vi "JamesPIDTEST.vi"() -> ()   [LabVIEW 2014]
uses:
  <vilib>/Rock Robotics/WPI/Solenoid/WPI_SolenoidValue.ctl
  Robot Global Data.vi
  <vilib>/addons/control/pid/NI_PID_pid.lvlib
  <vilib>/addons/control/pid/pid.llb/PID Advanced (DBL).vi
panel:
  out "Setpoint":dbl
  in  "setpoint range":cluster{"setpoint high":dbl, "setpoint low":dbl}={"setpoint high"=100.0, "setpoint low"=0.0}
  out "output":dbl format="%.2f"
  out "Brake":bool
  in  "proportional gain (Kc)":dbl step=0.01
  in  "integral time (Ti, min)":dbl step=0.01
  in  "derivative time (Td, min)":dbl step=0.01
  in  "dt (s)":dbl=-1.0 format="%.3f"
  in  "SetPoint":dbl(slide) scale=3.7..4.5
  out "dx/dt":dbl format="%.3f"
  out "Grabber":bool
  out "Turn on Brake":bool
  out "Delay?":bool
  out "VoltageDiff Valid?":bool
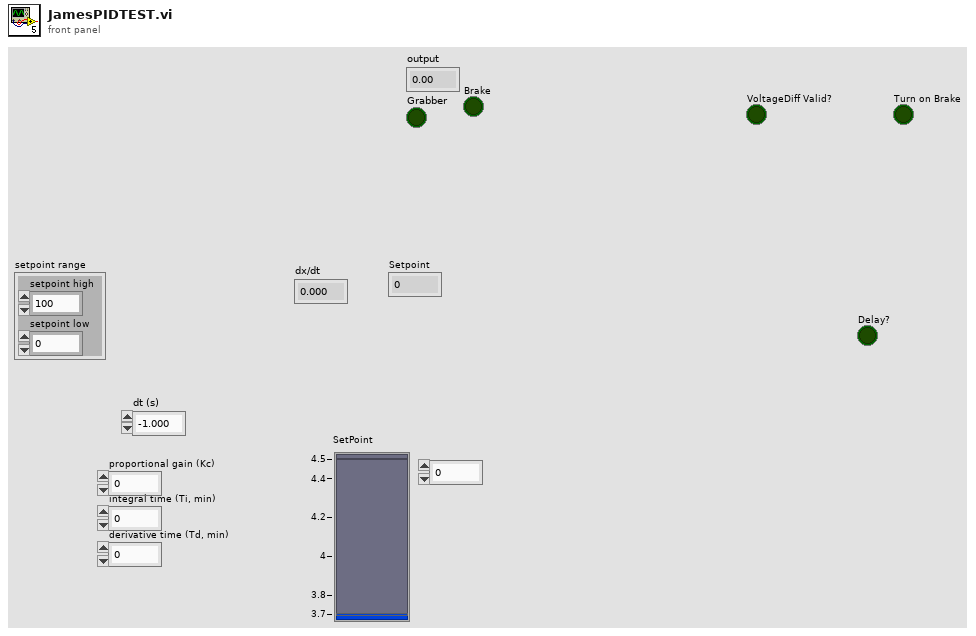
[diagram p1: front panel]
types:
  T1 = typedef "WPI_SolenoidDevRef.ctl" = cluster{"DevStatus":errorcluster, "Pneumatics Control Module":u8, "Forward Solenoid Channel":T2, "Reverse Solenoid Channel":T2}
  T2 = typedef "WPI_SolenoidChannel.ctl" = enum8{"Solenoid 0", "Solenoid 1", "Solenoid 2", "Solenoid 3", "Solenoid 4", "Solenoid 5", "Solenoid 6", "Solenoid 7", "Invalid"}
  T3 = typedef "WPI_MotorControlDeviceRef.ctl" = cluster{"DeviceStatus":errorcluster, "Type":T4, "PWM":cluster{"Controller":T5, "PWM Channel":T6, "DeadBand":T7}, "CAN":cluster{"Device Number":u8, "Control Mode":T8, "Semaphore":T9, "Max Vout":dbl, "TalonSRX Control Mode":T10}, "Invert":bool, "TransformRef":T11, "InvTransformRef":T11}
  T4 = typedef "WPI_MotorControlType.ctl" = enum16{"PWM", "CAN", "CANTalonSRX"}
  T5 = typedef "FPGA_TypedefDigitalModule.ctl" = enum16{"Controller 1"}
  T6 = typedef "FPGA_DIOPWMChannel.ctl" = enum8{"PWM 0", "PWM 1", "PWM 2", "PWM 3", "PWM 4", "PWM 5", "PWM 6", "PWM 7", "PWM 8", "PWM 9", "PWM MXP 0", "PWM MXP 1", "PWM MXP 2", "PWM MXP 3", "PWM MXP 4", "PWM MXP 5", "PWM MXP 6", "PWM MXP 7", "PWM MXP 8", "PWM MXP 9", "Invalid"}
  T7 = typedef "WPI_PWMDeadband.ctl" = cluster{"Name":string, "maxPositivePwm":i32, "minPositivePwm":i32, "centerPwm":i32, "maxNegativePwm":i32, "minNegativePwm":i32, "angularRange":u16}
  T8 = typedef "WPI_CANJaguar_ControlMode.ctl" = enum8{"Percent VBus", "Current", "Speed", "Position", "Voltage"}
  T9 = typedef "Semaphore RefNum" = refnum<k1>
  T10 = typedef "WPI_CANTalonSRX_APIControlMode.ctl" = enum8{"Percent VBus", "Speed", "Position", "Slave", "Unchanged / Invalid"}
  T11 = typedef "WPI_PWMTransform_ConPane.ctl" = refnum<vi>
  T12 = typedef "WPI_SolenoidValue.ctl" = enum16{"Off", "On", "Forward", "Reverse"}
  T13 = cluster{"proportional gain (Kc)":dbl, "integral time (Ti, min)":dbl, "derivative time (Td, min)":dbl}
  T14 = cluster{"Motor Speed":dbl, "Grabber":bool, "Go Up a Level":bool, "Go Down a Level":bool}
  T15 = cluster{"Front Right Motor":dbl, "Front Left Motor":dbl, "Rear Right Motor":dbl, "Rear Left Motor":dbl, "Current Heading":dbl, "Tote lift Up":bool, "Feeders Running":bool, "Pressure In Tank":dbl, "Image Data":string}
  T16 = cluster{"String Potentiometer":dbl, "Setpoint":dbl, "Level":sgl}
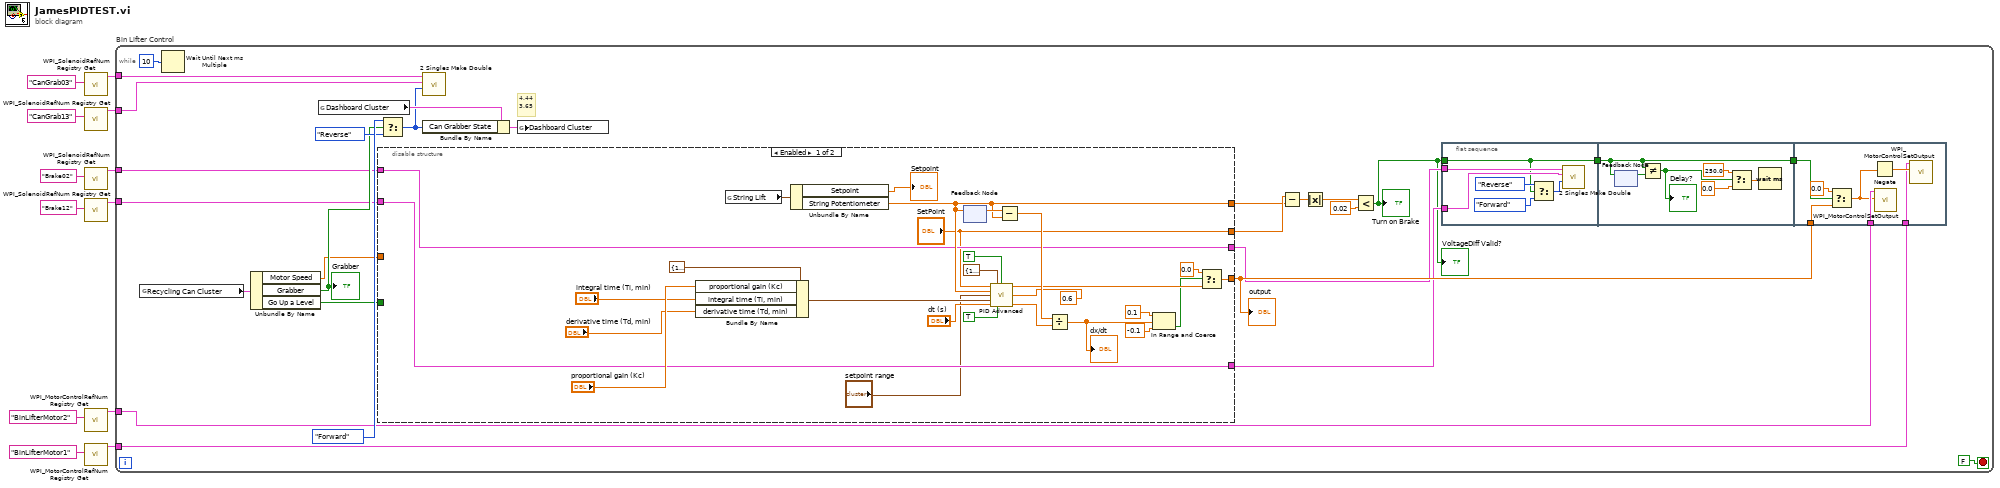
[diagram p0: block diagram]
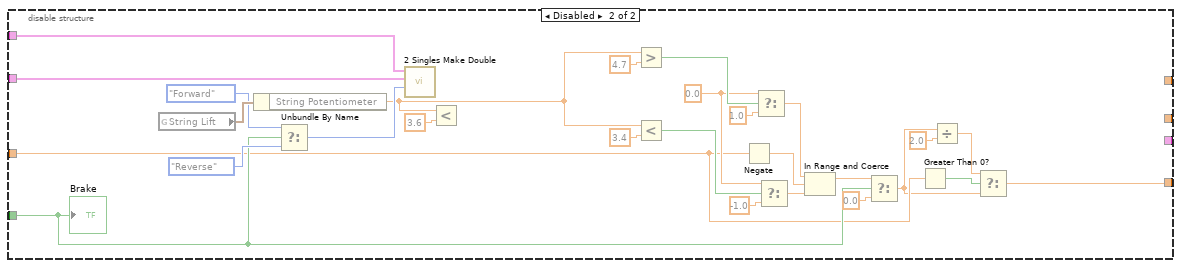
[diagram p2: hidden frame]
diagram:
  n1 = call <vilib>:"WPI_SolenoidRefNum Registry Get.vi"("refnum name"="CanGrab03") -> ("SolenoidDevRef"=w6:T1)  [unwired: 9 in, 1 out]
  n2 = call <vilib>:"WPI_SolenoidRefNum Registry Get.vi"("refnum name"="CanGrab13") -> ("SolenoidDevRef"=w5:T1)  [unwired: 9 in, 1 out]
  n3 = call <vilib>:"WPI_SolenoidRefNum Registry Get.vi"("refnum name"="Brake02") -> ("SolenoidDevRef"=w3:T1)  [unwired: 9 in, 1 out]
  n4 = call <vilib>:"WPI_SolenoidRefNum Registry Get.vi"("refnum name"="Brake12") -> ("SolenoidDevRef"=w2:T1)  [unwired: 9 in, 1 out]
  n5 = call <vilib>:"WPI_MotorControlRefNum Registry Get.vi"("refnum name"="BinLifterMotor2") -> ("MotorControlDevRef"=w4:T3)  [unwired: 9 in, 1 out]
  n6 = call <vilib>:"WPI_MotorControlRefNum Registry Get.vi"("refnum name"="BinLifterMotor1") -> ("MotorControlDevRef"=w1:T3)  [unwired: 9 in, 1 out]
  n7 = while "Bin Lifter Control" {
    tunnel: w4 -> [w34]
    tunnel: w1 -> [w33]
    tunnel: w5 -> [w29]
    tunnel: w6 -> [w30]
    tunnel: w3 -> [w25]
    tunnel: w2 -> [w24]
    stop <- FALSE stop-if-true
    # "4.44\n3.65"
    n8 = global read "Robot Global Data.vi" "Recycling Can Cluster"() -> (w39:T14)
    n9 = Wait Until Next ms Multiple(millisecond multiple=u32 10) -> ()  [unwired: 1 out]
    n10 = Unbundle By Name(w39) -> ("Motor Speed"=w27:dbl, "Grabber"=w31:bool, "Go Up a Level"=w26:bool)
    "Grabber" <- w31
    n11 = global read "Robot Global Data.vi" "Dashboard Cluster"() -> (w35:T15)
    n12 = disable-structure shown="Enabled" {
      disable-tunnel: [w61 w89] -> w21
      disable-tunnel: w27 -> [_ w92]
      disable-tunnel: w26 -> [_ w97]
      disable-tunnel: w25 -> [w70 w99]
      disable-tunnel: w24 -> [w69 w98]
      disable-tunnel: ["SetPoint" _] -> w23
      disable-tunnel: [w71 _] -> w22
      disable-tunnel: [w70 _] -> w20
      disable-tunnel: [w69 _] -> w19
      frame Enabled {
        n13 = Bundle By Name(cluster=T13 {"proportional gain (Kc)"=1.0, "integral time (Ti, min)"=0.01, "derivative time (Td, min)"=0.0} ("PID gains"), "proportional gain (Kc)"="proportional gain (Kc)", "integral time (Ti, min)"="integral time (Ti, min)", "derivative time (Td, min)"="derivative time (Td, min)") -> (w68:T13)
        n14 = global read "Robot Global Data.vi" "String Lift"() -> (w80:T16)
        n15 = Unbundle By Name(w80) -> ("Setpoint"=→"Setpoint":dbl, "String Potentiometer"=w71:dbl)
        n16 = feedback-in #1(w71) -> ()
        n17 = feedback #1() -> (w79:dbl)  [unwired: 1 in]
        n18 = call-poly <vilib>:"PID Advanced.vi"("setpoint"="SetPoint", "output range"=cluster{"output high":dbl, "output low":dbl} {"output high"=1.0, "output low"=-1.0}, "auto? (T)"=TRUE, "process variable"=w71, "setpoint range"="setpoint range", "alpha"=0.6, "PID gains"=w68, "dt (s)"="dt (s)", "reinitialize? (F)"=TRUE ("autotune? (F)")) -> ("output"=w74:dbl, "dt out (s)"=w78:dbl)  [unwired: 5 in]
        n19 = Subtract(x=w79, y=w71) -> (x-y=w77:dbl)
        n20 = Divide(x=w77, y=w78) -> (x/y=w72:dbl)
        "dx/dt" <- w72
        n21 = In Range and Coerce(upper limit=0.1, x=w72, lower limit=-0.1) -> (In Range?=w60:bool)  [unwired: 1 out]
        n22 = Select(t=0.0, s=w60, f=w74) -> (s? t:f=w61:dbl)
      }
      frame Disabled {
        w105 = 0.0 ("t")
        n23 = global read "Robot Global Data.vi" "String Lift"() -> (w113:T16)
        n24 = Unbundle By Name(w113) -> ("String Potentiometer"=w95:dbl)
        n25 = Select(t=WPI_SolenoidValue."Forward" ("Value"), s=w97, f=WPI_SolenoidValue."Reverse" ("Value")) -> (s? t:f=w100:T12)
        n26 = call "2 Singles Make Double.vi"("Value"=w100, "Reverse In"=w98, "Forward In"=w99) -> ()  [unwired: 7 in, 2 out]
        n27 = Less?(x=w95, y=3.6) -> ()  [unwired: 1 out]
        n28 = Greater?(x=w95, y=4.7) -> (0:w110:bool)
        n29 = Less?(x=w95, y=3.4) -> (x < y?=w107:bool)
        n30 = Negate(x=w92) -> (-x=w103:dbl)
        n31 = Select(t=w105, s=w110, f=1.0) -> (s? t:f=w109:dbl)
        n32 = Select(t=w105, s=w107, f=-1.0) -> (s? t:f=w108:dbl)
        n33 = In Range and Coerce(upper limit=w109, x=w103, lower limit=w108) -> (coerced(x)=w88:dbl)  [unwired: 1 out]
        n34 = Select(t=w88, s=w97, f=0.0 ("t")) -> (s? t:f=w91:dbl)
        n35 = Greater Than 0?(x=w92) -> (x > 0?=w94:bool)
        n36 = Divide(x=w91, y=2.0) -> (x/y=w93:dbl)
        n37 = Select(t=w93, s=w94, f=w91) -> (s? t:f=w89:dbl)
        "Brake" <- w97
      }
    }
    "output" <- w21
    n38 = Select(t=WPI_SolenoidValue."Forward" ("Value"), s=w31, f=WPI_SolenoidValue."Reverse" ("Value")) -> (s? t:f=w28:T12)
    n39 = call "2 Singles Make Double.vi"("Value"=w28, "Reverse In"=w29, "Forward In"=w30) -> ()  [unwired: 7 in, 2 out]
    n40 = Bundle By Name(cluster=w35, "Can Grabber State"=w28) -> (w36:T15)
    n41 = global write "Robot Global Data.vi" "Dashboard Cluster"(w36) -> ()
    n42 = Subtract(x=w23, y=w22) -> (x-y=w16:dbl)
    n43 = Absolute Value(x=w16) -> (abs(x)=w15:dbl)
    n44 = Less?(x=w15, y=0.02) -> (x < y?=w13:bool)
    "Turn on Brake" <- w13
    "VoltageDiff Valid?" <- w13
    n45 = flat-sequence {
      tunnel: w13 -> [w41]
      tunnel: w20 -> [w44]
      tunnel: w19 -> [w43]
      tunnel: [w41] -> w18
      tunnel: w18 -> [w47]
      tunnel: [w47] -> w17
      tunnel: w34 -> [w59]
      tunnel: w17 -> [w57]
      tunnel: w21 -> [w56]
      tunnel: w33 -> [w53]
      frame #0 {
        n46 = Select(t=WPI_SolenoidValue."Reverse" ("Value"), s=w41, f=WPI_SolenoidValue."Forward" ("Value")) -> (s? t:f=w42:T12)
        n47 = call "2 Singles Make Double.vi"("Value"=w42, "Reverse In"=w43, "Forward In"=w44) -> ()  [unwired: 7 in, 2 out]
      }
      frame #1 {
        n48 = feedback #2() -> (w48:bool)  [unwired: 1 in]
        n49 = feedback-in #2(w47) -> ()
        n50 = Not Equal?(x=w47, y=w48) -> (x != y?=w52:bool)
        "Delay?" <- w52
        n51 = Select(t=250.0, s=w52, f=0.0) -> (s? t:f=w51:dbl)
        n52 = Wait (ms)(milliseconds to wait=w51) -> ()  [unwired: 1 out]
      }
      frame #2 {
        n53 = Select(t=0.0, s=w57, f=w56) -> (s? t:f=w54:dbl)
        n54 = Negate(x=w54) -> (-x=w55:dbl)
        n55 = call <vilib>:"WPI_MotorControlSetOutput.vi"("Output"=w54, "MotorControlDevRef"=w59) -> ()  [unwired: 7 in, 3 out]
        n56 = call <vilib>:"WPI_MotorControlSetOutput.vi"("Output"=w55, "MotorControlDevRef"=w53) -> ()  [unwired: 7 in, 3 out]
      }
    }
  }
